vi "AxB.vi"(1 "B":u8, 2 "A":u8) -> (0 "Numeric":u8)   [LabVIEW 2017]
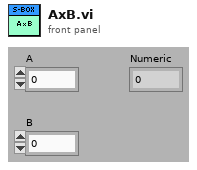
[diagram p1: front panel]
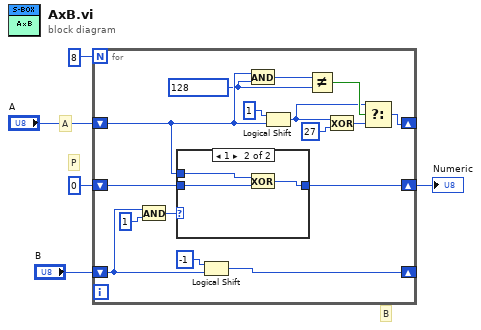
[diagram p0: block diagram]
diagram:
  # "P"
  # "B"
  # "A"
  n1 = for {
    N: 8 -> [_]
    shift-right: [w9] -> _
    shift-left: "A" -> [w19]
    shift-right: [w8] -> _
    shift-left: "B" -> [w6]
    shift-right: [w7] -> w4
    shift-left: u8 0 -> [w20]
    w16 = u8 128 ("y")
    n2 = And(x=w6, y=u8 1) -> (x .and. y?=w10:u8)
    n3 = case shown="1" w10 {
      tunnel: w20 -> [w22 w25]
      tunnel: w19 -> [_ w24]
      tunnel: [w22 w23] -> w7
      frame 0, Default {
      }
      frame 1 {
        n4 = Exclusive Or(1:w25, 2:w24) -> (0:w23:u8)
      }
    }
    n5 = Logical Shift(y=i8 -1, x=w6) -> (x << y=w8:u8)
    n6 = And(x=w19, y=w16) -> (x .and. y?=w17:u8)
    n7 = Logical Shift(y=i8 1, x=w19) -> (x << y=w14:u8)
    n8 = Not Equal?(x=w17, y=w16) -> (x != y?=w15:bool)
    n9 = Exclusive Or(1:u8 27 ("y"), 2:w14) -> (0:w13:u8)
    n10 = Select(t=w14, s=w15, f=w13) -> (s? t:f=w9:u8)
  }
  "Numeric" <- w4
